vi "TalonFX_SetPosition.vi"(6 "timeoutSeconds":dbl=0.05, 10 "Position":dbl, 11 "DeviceReference":T1) -> ()   [LabVIEW 2023]
uses:
  Users/Cory/Documents/PhoenixPro-LabVIEW-Generation/controls/DeviceReference.ctl
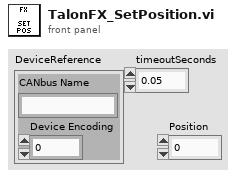
[diagram p1: front panel]
types:
  T1 = typedef "DeviceReference.ctl" = cluster{"CANbus Name":string, "Device Encoding":u32}
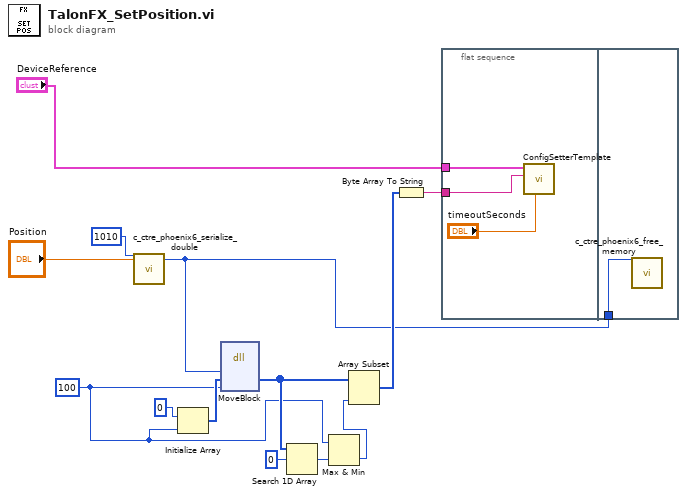
[diagram p0: block diagram]
diagram:
  w2 = i64 100 ("size")
  n1 = call <vilib>:"c_ctre_phoenix6_serialize_double.vi"("Numeric 2"=1010, "Numeric 3"="Position") -> ("Numeric 4"=w6:u32)  [unwired: 24 in, 1 out]
  n2 = Initialize Array(u8 0 ("element"), w2) -> (w13:u8[])
  n3 = dll-call lib="LabVIEW" fn="MoveBlock"("ps"=w6, "pd"=w13, "size"=w2) -> ("pd"=w5:u8[])  [unwired: 6 in, 2 out]
  n4 = Search 1D Array(1D array=w5, element=u8 0) -> (index of element=w3:i32)  [unwired: 1 in]
  n5 = Max & Min(x=w2, y=w3) -> (min(x,y)=w1:i64)  [unwired: 1 out]
  n6 = Array Subset(array=w5, length=w1) -> (w11:u8[])  [unwired: 1 in]
  n7 = Byte Array To String(unsigned byte array=w11) -> (string=w9:string)
  n8 = flat-sequence {
    tunnel: w9 -> [w15]
    tunnel: "DeviceReference" -> [w14]
    tunnel: w6 -> [w17]
    frame #0 {
      n9 = call <vilib>:"ConfigSetterTemplate.vi"("timeoutSeconds"="timeoutSeconds", "Configs"=w15, "DeviceReference"=w14) -> ()  [unwired: 8 in, 1 out]
    }
    frame #1 {
      n10 = call <vilib>:"c_ctre_phoenix6_free_memory.vi"("Numeric 3"=w17) -> ()  [unwired: 25 in, 2 out]
    }
  }
